vi "Discipline PXI_Clk10 to 1588 and Gen PPS.vi"() -> ()   [LabVIEW 2016]
doc: "Description:\nThis VI demonstrates disciplining the PXI_Clk10 using a single board disciplining capable Timing module.\n\nHW Requirements:\nSingle board disciplining capable System Timing module in the System Timing Slot of the PXI chassis\n(see File » VI Properties » Documentation for more information)"
uses:
  <instrlib>/niSync/niSync.llb/niSync Create Clock (Frequency).vi
  <instrlib>/niSync/niSync.llb/niSync Initialize (IVI).vi
  <instrlib>/niSync/niSync.llb/niSync Set Time Reference (1588 Ordinary Clock).vi
panel:
  in  "Desired Clock Frequency (Hz)":u32=1
  out "Offset from Time Reference":dbl format="%#_p"
  out "Is Time Reference Present?":bool
  in  "6682 Device Name":refnum<k15>="PXI1Slot2"
  # "Discipline PXI_Clk10 to 1588 and Gen PPS.viOverview: Demonstrates disciplining PXI_Clk10 using a single board disciplining capable time-based device.\nRequirements: LabVIEW Full Development System, NI-Sync 3.4 or later, single board disciplining capable time-based device.\nInstructions:\n1. Ensure the time-based device is in the system Timing slot.\n2. Set the desired time reference for the time-based device.\n    Note:  You do not need to specify a value for IRIG Type unless Time Reference is set to IRIG.\n    Note:  You do not need to specify a value for Time Reference Terminal  unless Time Reference is set to IRIG or PPS.\n3. Run the VI."
  # "Time Reference Information"
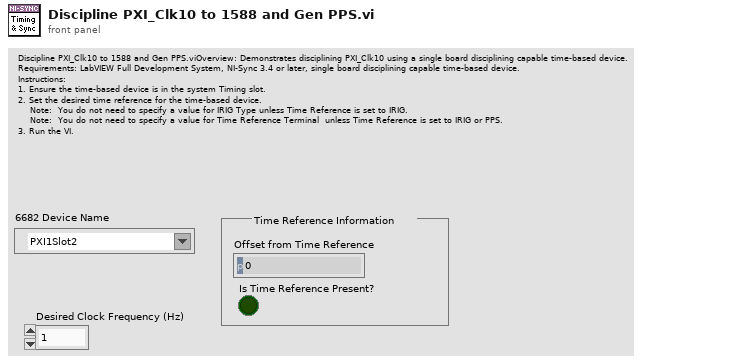
[diagram p1: front panel]
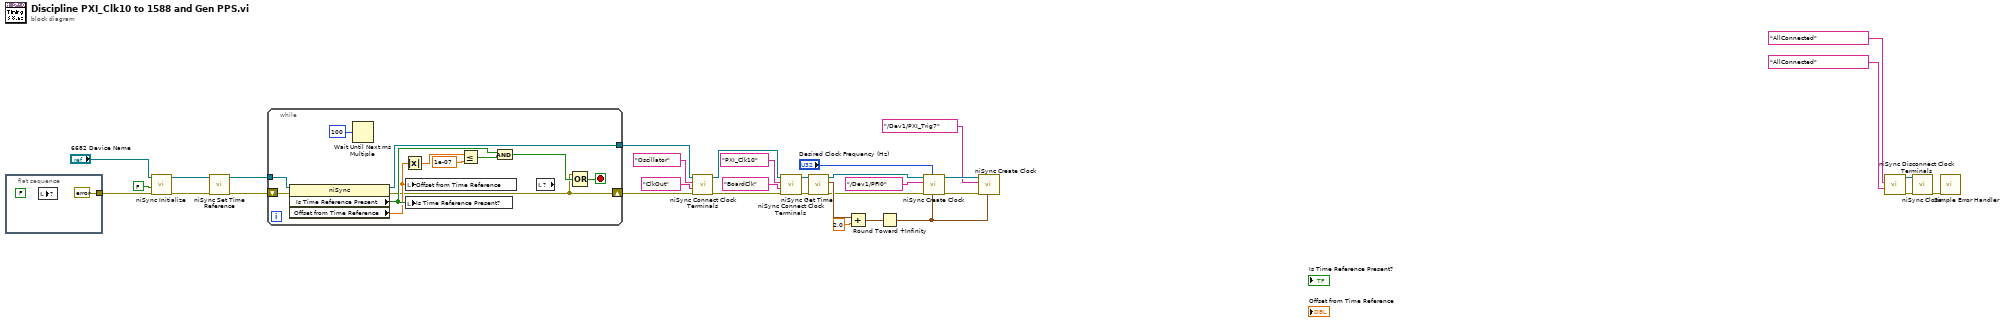
[diagram p0: block diagram]
diagram:
  n1 = flat-sequence {
    tunnel: [errorcluster {"status"=FALSE, "code"=0, "source"=""} ("error in (no error)")] -> w2
    frame #0 {
      (unwired) FALSE ("stop")
      n2 = local read item#-1() -> ()  [unwired: 1 in]
    }
  }
  n3 = call-poly <instrlib>:"niSync Initialize.vi"("error in (no error)"=w2, "reset device (F)"=FALSE ("reset device (False)"), "resource name"="6682 Device Name") -> ("error out"=w25:errorcluster, "instrument handle out"=w24:refnum<k15>)  [unwired: 7 in]
  n4 = call-poly <instrlib>:"niSync Set Time Reference.vi"("error in (no error)"=w25, "instrument handle"=w24) -> ("error out"=w4:errorcluster, "instrument handle out"=w6:refnum<k15>)  [unwired: 8 in]
  n5 = while {
    tunnel: w6 -> [w46]
    tunnel: [w45] -> w5
    shift-right: [w35] -> w3
    shift-left: w4 -> [w44]
    stop <- w37 stop-if-true
    n6 = property class="niSync"(reference=w46, error in=w44) -> (reference out=w45:refnum<k15>, error out=w35:errorcluster, "Is Time Reference Present"=w40:bool, "Offset from Time Reference"=w39:dbl)
    n7 = Wait Until Next ms Multiple(millisecond multiple=u32 100) -> ()  [unwired: 1 out]
    n8 = Absolute Value(x=w39) -> (abs(x)=w43:dbl)
    n9 = local write "Offset from Time Reference"(w39) -> ()
    n10 = local write "Is Time Reference Present?"(w40) -> ()
    n11 = Less Or Equal?(x=w43, y=1e-07) -> (x <= y?=w42:bool)
    n12 = Compound Arithmetic op=AND(w40, w42) -> (w36:bool)
    n13 = local read item#-1() -> ()  [unwired: 1 out]
    n14 = Compound Arithmetic op=OR(w35, w36) -> (w37:bool)  [unwired: 1 in]
  }
  n15 = call <instrlib>:"niSync Connect Clock Terminals.vi"("error in (no error)"=w3, "destination terminal"="ClkOut", "source terminal"="Oscillator", "instrument handle"=w5) -> ("error out"=w31:errorcluster, "instrument handle out"=w30:refnum<k15>)  [unwired: 6 in]
  n16 = call <instrlib>:"niSync Connect Clock Terminals.vi"("error in (no error)"=w31, "destination terminal"="BoardClk", "source terminal"="PXI_Clk10", "instrument handle"=w30) -> ("error out"=w13:errorcluster, "instrument handle out"=w14:refnum<k15>)  [unwired: 6 in]
  n17 = call <instrlib>:"niSync Get Time.vi"("error in (no error)"=w13, "instrument handle"=w14) -> ("error out"=w17:errorcluster, "time"=w19:timestamp, "instrument handle out"=w18:refnum<k15>)  [unwired: 5 in]
  n18 = Add(x=w19, y=2.0) -> (x+y=w15:timestamp)
  n19 = Round Toward +Infinity(x=w15) -> (ceil(x): smallest int >= x=w7:timestamp)
  n20 = call-poly <instrlib>:"niSync Create Clock.vi"("start time"=w7, "frequency"="Desired Clock Frequency (Hz)", "error in (no error)"=w17, "terminal"=tag "/Dev1/PFI0", "instrument handle"=w18) -> ("error out"=w9:errorcluster, "instrument handle out"=w10:refnum<k15>)  [unwired: 3 in, 2 out]
  n21 = call-poly <instrlib>:"niSync Create Clock.vi"("start time"=w7, "error in (no error)"=w9, "terminal"=tag "/Dev1/PXI_Trig7", "instrument handle"=w10) -> ()  [unwired: 4 in, 4 out]
  n22 = call <instrlib>:"niSync Disconnect Clock Terminals.vi"("destination terminal"="AllConnected", "source terminal"="AllConnected") -> ("error out"=w21:errorcluster, "instrument handle out"=w20:refnum<k15>)  [unwired: 8 in]
  n23 = call <instrlib>:"niSync Close.vi"("error in (no error)"=w21, "instrument handle"=w20) -> ("error out"=w1:errorcluster)  [unwired: 9 in]
  n24 = call <vilib>:"Simple Error Handler.vi"("error in (no error)"=w1) -> ()  [unwired: 4 in, 5 out]
